vi "Set Lifecycle State.vi"(8 "error in (no error)":errorcluster, 10 "Lifecycle State":T1, 11 "Process In":refnum<class "Debug View.lvclass">) -> (0 "error out":errorcluster, 3 "Process Out":refnum<class "Debug View.lvclass">)   [LabVIEW 2020]
uses:
  Debug View.lvclass
  Public/Lifecycle/Lifecycle State.ctl
  Debug View.lvclass/Debug View.ctl
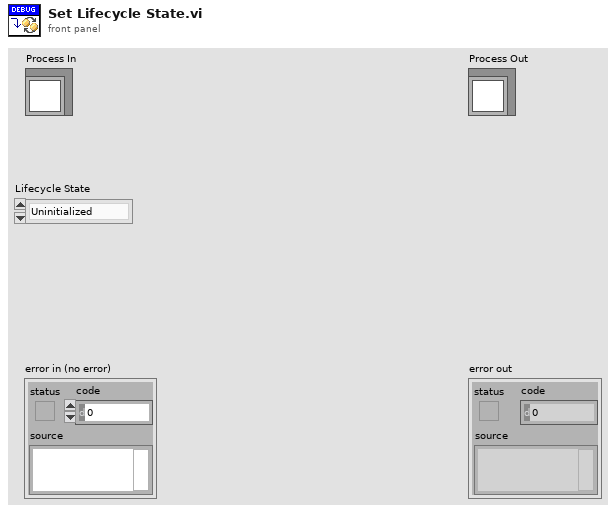
[diagram p1: front panel]
types:
  T1 = typedef "Lifecycle State.ctl" = enum16{"Uninitialized", "Initialized", "Started", "Running", "Stopped", "Finished"}
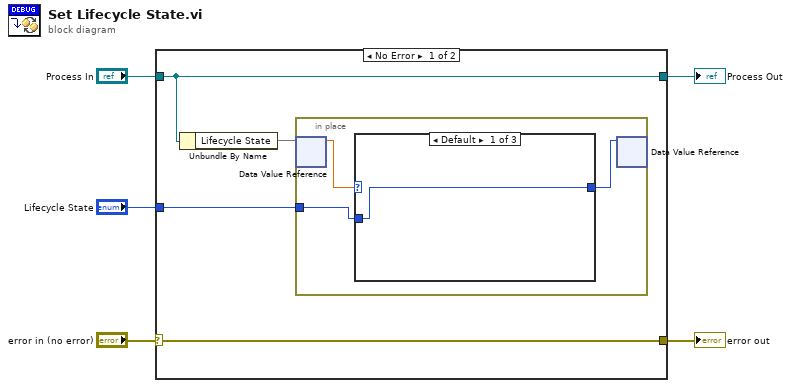
[diagram p0: block diagram]
diagram:
  n1 = case shown="No Error" "error in (no error)" {
    selector: "error in (no error)" -> [w7 w25]
    tunnel: "Process In" -> [w6 w24]
    tunnel: "Lifecycle State" -> [w8 _]
    tunnel: [w7 w25] -> w2
    tunnel: [w6 w24] -> w1
    frame No Error {
      n2 = Unbundle By Name(w6) -> ("Lifecycle State"=w9)
      n3 = in-place {
        in-place-border: w8 -> [w12]
        n4 = in-place-dvr #1(w9) -> (w11:dbl)  [unwired: 1 out]
        n5 = case shown="Default" w11 {
          selector: w11 -> [_ w14 w19]
          tunnel: w12 -> [w13 w16 w21]
          tunnel: [w13 w15 w20] -> w10
          frame Default {
          }
          frame 3 {
            n6 = case shown="Default" w16 {
              selector: w16 -> [w17 _]
              tunnel: [w17 w18] -> w15
              tunnel: w14 -> [_ w18]
              frame Default {
              }
              frame "Started" {
              }
            }
          }
          frame 4 {
            n7 = case shown="Default" w21 {
              selector: w21 -> [w22 _]
              tunnel: [w22 w23] -> w20
              tunnel: w19 -> [_ w23]
              frame Default {
              }
              frame "Running" {
              }
            }
          }
        }
        n8 = in-place-dvr #1(w10) -> ()  [unwired: 2 out]
      }
    }
    frame Error {
    }
  }
  "error out" <- w2
  "Process Out" <- w1
